vi "Configure VNA - Dual Port Instrument Handle.vi"(7 "VNA Instrument Handle Array":refnum<k15>[](array[refnum]), 8 "error in (no error)":errorcluster, 9 "Pins":string[](array[string]), 10 "Calibration File Paths":path[](array[path]), 11 "Semiconductor Module Context":T2) -> (0 "error out":errorcluster, 3 "VNA Measurement Parameters Out":T1)   [LabVIEW 2013]
uses:
  <vilib>/NI_TestStand_SemiconductorModule/NI_TestStand_Semiconductor_Module.lvlibp/PinMap/General/SemiconductorModuleContext.ctl
  VNAs Measurement Parameters.ctl
  <vilib>/NI_TestStand_SemiconductorModule/NI_TestStand_Semiconductor_Module.lvlibp/PinMap/General/NIInstrumentTypeIDs.ctl
  <instrlib>/niVNA/niVNA.llb/niVNA Load Calibration And Configuration Data From File.vi
  Pin Map API/VNA Custom Instrument.lvlib
  <vilib>/NI_TestStand_SemiconductorModule/NI_TestStand_Semiconductor_Module.lvlibp
panel:
  out "Averaging And Smoothing:Averaging Count":i32
  out "Sweep:Sweep Frequency Start":dbl
  out "Sweep:Sweep Frequency Stop":dbl
  out "instrument handle":refnum<k15>
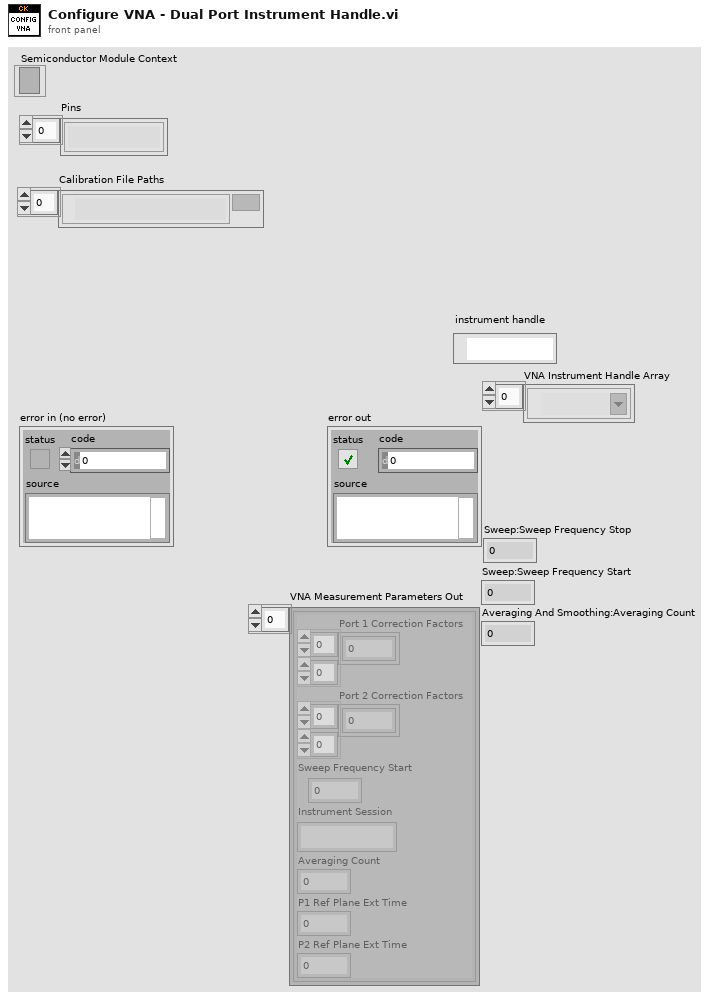
[diagram p1: front panel]
types:
  T1 = typedef "VNAs Measurement Parameters.ctl" = cluster{"Port 1 Correction Factors":cdb[][], "Port 2 Correction Factors":cdb[][], "Sweep Frequency Start":dbl, "Instrument Session":string, "Averaging Count":i32, "P1 Ref Plane Ext Time":dbl, "P2 Ref Plane Ext Time":dbl}[]
  T2 = typedef "NI_TestStand_Semiconductor_Module.lvlibp/SemiconductorModuleContext.ctl" = refnum<k7>
  T3 = typedef "NI_TestStand_Semiconductor_Module.lvlibp/NIInstrumentTypeIDs.ctl" = string
  T4 = typedef "Two Port Corerction Factors.ctl" = cluster{"Forward e00":cdb[], "Forward e11":cdb[], "Forward e10e01":cdb[], "Forward e30":cdb[], "Forward e22":cdb[], "Forward e10e32":cdb[], "Reverse e33":cdb[], "Reverse e22 ":cdb[], "Reverse e23e32":cdb[], "Reverse e03":cdb[], "Reverse e11":cdb[], "Reverse e23e01":cdb[]}
  T5 = typedef "VNA Measurement Parameters2.ctl" = cluster{"Port 1 Correction Factors":cdb[][], "Port 2 Correction Factors":cdb[][], "Sweep Frequency Start":dbl, "Instrument Session":string, "Averaging Count":i32, "P1 Ref Plane Ext Time":dbl, "P2 Ref Plane Ext Time":dbl}
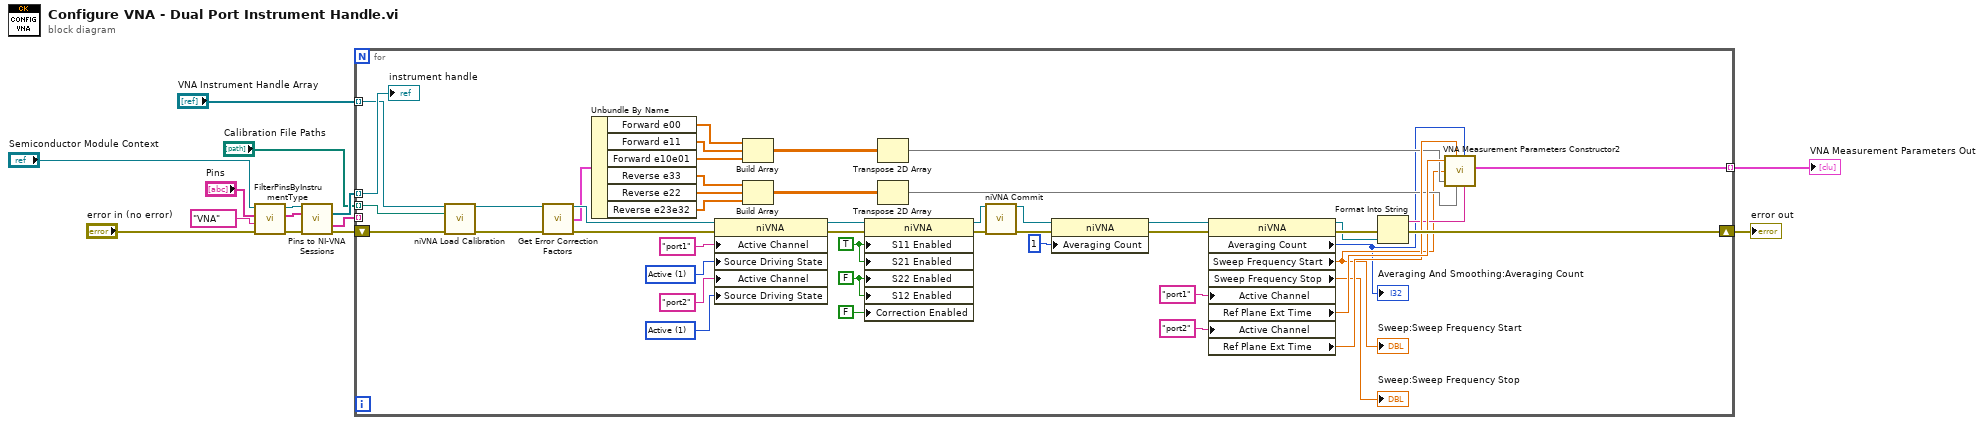
[diagram p0: block diagram]
diagram:
  n1 = call <vilib>:"FilterPinsByInstrumentType.vi"("error in (no error)"="error in (no error)", "Instrument Type Id"=T3 "VNA", "Pins"="Pins", "Semiconductor Module Context"="Semiconductor Module Context") -> ("error out"=w12:errorcluster, "Filtered Pins"=w11:string[], "Semiconductor Module Context Out"=w10:T2)  [unwired: 5 in]
  n2 = call "Pins to NI-VNA Sessions.vi"("Semiconductor Module Context"=w10, "Pins"=w11, "error in (no error)"=w12) -> ("Instrument Sessions"=w14:refnum<k15>[], "Channel Lists"=w13:string[], "error out"=w4:errorcluster)  [unwired: 8 in, 2 out]
  n3 = for {
    tunnel: w14 -> [w24] mode=indexing
    tunnel: "Calibration File Paths" -> [w60] mode=indexing
    tunnel: w13 -> [_] mode=indexing
    shift-right: [w32] -> w3
    shift-left: w4 -> [w61]
    tunnel: [w30] -> w2 mode=indexing
    tunnel: "VNA Instrument Handle Array" -> [w23] mode=indexing
    w51 = FALSE ("Sweep:S11 Enabled")
    w52 = TRUE ("Sweep:S11 Enabled")
    w46 = 1 items=["Automatic", "Active", "Inactive"] ("Individual Sources/Receiver:Source Driving State")
    w56 = 1 items=["Automatic", "Active", "Inactive"] ("Individual Sources/Receiver:Source Driving State")
    n4 = call-poly <instrlib>:"niVNA Load Calibration.vi"("instrument handle"=w23, "file path"=w60, "error in"=w61) -> ("instrument handle out"=w59:refnum<k15>, "error out"=w58:errorcluster)  [unwired: 11 in]
    n5 = call "Get Error Correction Factors.vi"("instrument handle"=w59, "Error In"=w58) -> ("instrument handle out"=w48:refnum<k15>, "Two Port Correction Factors"=w36:T4, "Error Out"=w49:errorcluster)  [unwired: 11 in]
    n6 = Unbundle By Name(w36) -> ("Forward e00"=w44:cdb[], "Forward e11"=w43:cdb[], "Forward e10e01"=w42:cdb[], "Reverse e33"=w39:cdb[], "Reverse e22"=w40:cdb[], "Reverse e23e32"=w41:cdb[])
    n7 = property class="niVNA"(reference=w48, error in=w49, "Active Channel"="port1", "Source Driving State"=w56, "Active Channel"="port2", "Source Driving State"=w46) -> (reference out=w53:refnum<k15>, error out=w54:errorcluster)
    n8 = Build Array(w44, w43, w42) -> (w38:cdb[][])
    n9 = Build Array(w39, w40, w41) -> (w37:cdb[][])
    n10 = property class="niVNA"(reference=w53, error in=w54, "S11 Enabled"=w52, "S21 Enabled"=w52, "S22 Enabled"=w51, "S12 Enabled"=w51, "Correction Enabled"=FALSE ("Calibration Settings:Correction Enabled")) -> (reference out=w47:refnum<k15>, error out=w45:errorcluster)
    n11 = Transpose 2D Array(2D array=w38) -> (transposed array=w27:cdb[][])
    n12 = Transpose 2D Array(2D array=w37) -> (transposed array=w26:cdb[][])
    n13 = call <instrlib>:"niVNA Commit.vi"("instrument handle"=w47, "error in"=w45) -> ("instrument handle out"=w16:refnum<k15>, "error out"=w18:errorcluster)  [unwired: 12 in]
    n14 = property class="niVNA"(reference=w16, error in=w18, "Averaging Count"=1 ("Averaging And Smoothing:Averaging Count")) -> (reference out=w15:refnum<k15>, error out=w17:errorcluster)
    n15 = property class="niVNA"(reference=w15, error in=w17, "Active Channel"="port1", "Active Channel"="port2") -> (reference out=w31:refnum<k15>, error out=w33:errorcluster, "Averaging Count"=w19:i32, "Sweep Frequency Start"=w21:dbl, "Sweep Frequency Stop"=→"Sweep:Sweep Frequency Stop":dbl, "Ref Plane Ext Time"=w29:dbl, "Ref Plane Ext Time"=w28:dbl)
    "Sweep:Sweep Frequency Start" <- w21
    "Averaging And Smoothing:Averaging Count" <- w19
    n16 = Format Into String(error in=w33, w31) -> (resulting string=w25:string, error out=w32:errorcluster)  [unwired: 2 in]
    n17 = call "VNA Measurement Parameters Constructor2.vi"("P1 Ref Plane Ext Time"=w29, "P2 Ref Plane Ext Time"=w28, "Sweep Frequency Start"=w21, "Port 1 Correction Factors"=w27, "Port 2 Correction Factors"=w26, "Averaging Count"=w19, "Instrument Session"=w25) -> ("VNA Measurement Parameters Out"=w30:T5)  [unwired: 3 in]
    "instrument handle" <- w24
  }
  "error out" <- w3
  "VNA Measurement Parameters Out" <- w2
